vi "Legacy_ProdLight MainUI_controls_and_indicators.vi"() -> ()   [LabVIEW 2017]
uses:
  Ichor_Common/DataTypes/LocalSMDirect EvData--cluster.ctl
  Ichor_Common/DataTypes/LocalSMDirect EvData Mode Selection--enum.ctl
panel:
  in  "AbortSeq - NonLatchingCtrl":bool
  in  "LocalSMDirect EvData":T1
  in  "MoveTowardFast":bool caption="Move \nToward\nFast"
  in  "MoveToZero":bool caption="Move to \nZero"
  in  "MoveAwayFast":bool caption="Move \nAway Fast"
  in  "MoveToward":bool caption="Move \nToward (-)"
  in  "MoveAway":bool caption="Move \nAway (+)"
  out "Safety OK":bool
  in  "SystemError":bool
  out "Pos Err (cnts)":dbl
  out "MotorPos(in)":dbl caption="Motor Position (in)" format="%.3f"
  in  "StatusMsg":string caption="Status"
  in  "Weld Enable":bool caption="Weld Current\nSetpoint"
  out "JoggingTurntable":bool
  in  "JogTurntable":bool caption="Click and Hold"
  out "SeqLoaded":bool caption="Sequence Loaded"
  out "SeqAborted":bool caption="Sequence Aborted"
  in  "AbortSeq":bool
  in  "MotorCtrlLoop Enable":bool caption="Motor Pos\nLoop Ctrl"
  in  "Turntable Enable":bool caption="Turntable On"
  out "SeqRunning":bool
  in  "StartSeq":bool
  out "Sequence File":string
  in  "Tab Control":enum32{"Config", "Data", "Motor", "Seq"}(tab)
  in  "IgnoreMtrRspnsErr":bool caption="Ignore Motor\nResponse Error\nDuring Seq"
  in  "AVC ConfigUtility":bool caption="AVC Configuration\nUtility"
  in  "SamplingRate":dbl=1000.0 caption="Sampling\nRate"
  in  "NumSamples":i32=100 caption="Samples per\nAcquistion"
  in  "UpdateDAQSettings":bool
  in  "DAQ Rd & MtrSP Interval":u32
  in  "WriteLogFile Interval":u32
  in  "DAQDisplay Interval":i32
  out "DAQEnabled":bool
  in  "DAQEnDis":bool
  out "LogEnabled":bool
  in  "LogEnDis":bool
  out "TDMSEnabled":bool
  in  "TDMSEnDis":bool
  in  "PosCtlrSettings":bool caption="Position Ctlr\nRunTime Settings"
  out "MotorRspnsErr":bool caption="Motor Response\nError"
  out "TotalVgain":dbl caption="Total Ctlr\nVgain" format="%.3f"
  out "Motor SP":dbl caption="Computed Motor\nPos Chg (in)" format="%.3f"
  out "VoltageError":dbl caption="Voltage Error" format="%.3f"
  out "WeldTime":dbl caption="Weld Time (s)" format="%.2f"
  out "voltage fb":dbl caption="Voltage" format="%.3f"
  out "Current SP":dbl format="%.3f"
  out "Current fb":dbl caption="Current" format="%.3f"
  out "ProcessTime":dbl caption="Process Time (s)" format="%.2f"
  out "AVC Lockout":bool
  out "In Range?":bool
  out "VspOffset":dbl
  out "Volts and Current Chart":T3(graph)
  in  "GraphEnable":bool
  out "DAQ Latency":bool caption="Time has Elapsed"
  out "SeqList":i32(listbox) caption="Sequence"
  out "Step Comment":string
  in  "Turntable \nSpeed (RPM)":dbl(knob) scale=0.0..10.0
  out "Process Complete":bool caption="Time has Elapsed"
  out "Weld Profile Graph":cluster{dbl[], dbl[]}(graph)
  out "Weld Current Waveform Chart":dbl(graph)
  in  "Exit":bool
  # "Motor Controls"
  # "Right-Click to Load Sequence"
  # "Current Profile"
  # "Current Out (Trend Ref Only)"
  # "Configuration Panel"
  # "DAQ Settings"
  # "Run Time Data Panel"
  # "V & I Process Feedback"
  # "click to reset"
  # "Voltage FB (V)"
  # "Current FB (A)"
  # "Motor Pos (in)"
  # "Right-Click to Clear"
  # "Arc Voltage Control Production Lite System"
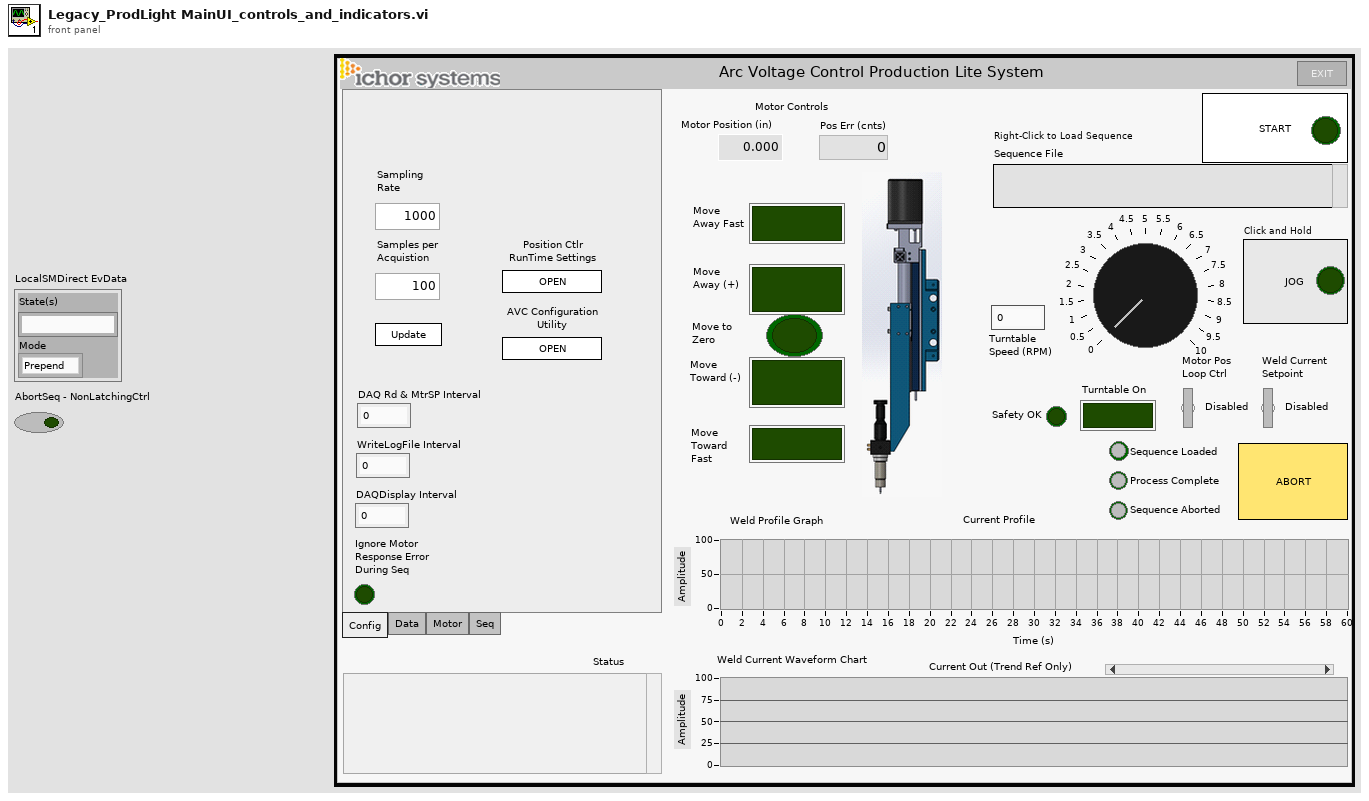
[diagram p1: front panel]
types:
  T1 = typedef "LocalSMDirect EvData--cluster.ctl" = cluster{"State(s)":string, "Mode":T2}
  T2 = typedef "LocalSMDirect EvData Mode Selection--enum.ctl" = enum16{"Prepend", "Append", "Replace"}
  T3 = cluster{"VoltageDyn":dbl, "CurrentDyn":dbl, "MotorV SP":dbl}
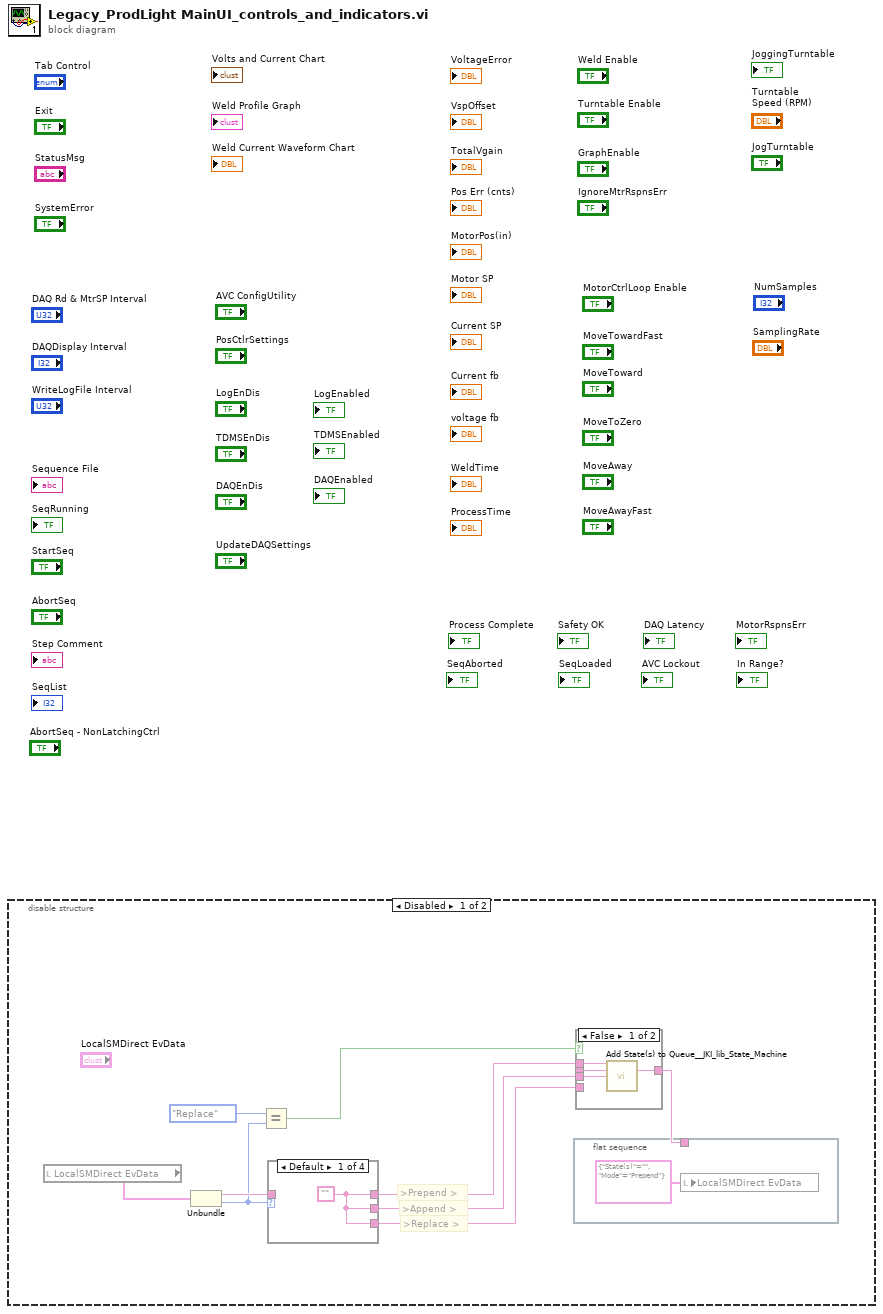
[diagram p0: block diagram]
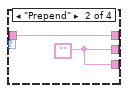
[diagram p3: hidden frame]
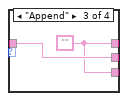
[diagram p4: hidden frame]
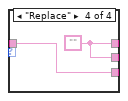
[diagram p5: hidden frame]
diagram:
  n1 = disable-structure shown="Disabled" {
    frame Disabled {
      # ">Replace >"
      # ">Append >"
      # ">Prepend >"
      n2 = local read "LocalSMDirect EvData"() -> (w1:T1)
      n3 = Unbundle(w1) -> ("State(s)"=w9:string, "Mode"=w8:T2)
      n4 = Equal?(x=LocalSMDirect_EvData_Mode_Selection--enum."Replace", y=w8) -> (x = y?=w6:bool)
      n5 = case shown="Default" w8 {
        tunnel: w9 -> [_ w19 w21 w23]
        tunnel: [w17 w19 w20 w22] -> w5
        tunnel: [w17 w18 w21 w22] -> w4
        tunnel: [w17 w18 w20 w23] -> w3
        frame Default {
          w17 = ""
        }
        frame "Prepend" {
          w18 = ""
        }
        frame "Append" {
          w20 = ""
        }
        frame "Replace" {
          w22 = ""
        }
      }
      n6 = flat-sequence {
        tunnel: w2 -> [_]
        frame #0 {
          n7 = local write "LocalSMDirect EvData"(T1 {"State(s)"="", "Mode"=enum."Prepend"} ("LocalSMDirect EvData")) -> ()
        }
      }
      n8 = case shown="False" w6 {
        tunnel: [w15 _] -> w10
        tunnel: [w14 w16] -> w2
        tunnel: w5 -> [w13 _]
        tunnel: w4 -> [w12 _]
        tunnel: w3 -> [_ w16]
        frame False {
          n9 = call <vilib>:"Add State(s) to Queue__JKI_lib_State_Machine.vi"("State(s) in Front (\"\")"=w13, "State(s) in (\"\")"=w15, "State(s) at Back (\"\")"=w12) -> ("States Out"=w14:string)  [unwired: 12 in]
        }
        frame True {
        }
      }
    }
    frame Enabled {
    }
  }
